vi "plotFrd.vi"(8 "error in (no error)":errorcluster, 9 "FRD-array":T1[](array[typedef]), 10 "Phase Graph Reference in":refnum<vi>, 11 "Magnitude Graph Reference in":refnum<vi>) -> (0 "error out":errorcluster, 2 "Phase Graph Reference out":refnum<vi>, 3 "Magnitude Graph Reference out":refnum<vi>)   [LabVIEW 2017]
uses:
  auto-sys-id/controls/FrdData.ctl
  <vilib>/Analysis/NI_AALPro.lvlib
panel:
  in  "Frequency Unit":enum16{"Hz", "rad/s"}(ring)
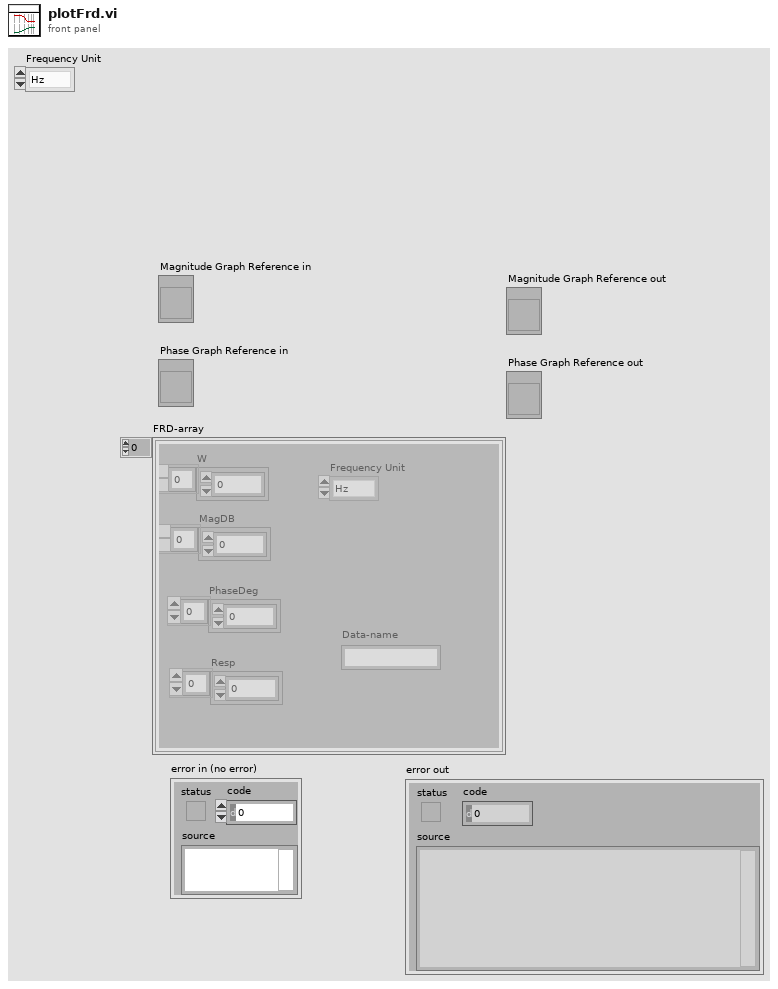
[diagram p1: front panel]
types:
  T1 = typedef "FrdData.ctl" = cluster{"Frequency Unit":enum16{"Hz", "rad/s"}, "W":dbl[], "MagDB":dbl[], "PhaseDeg":dbl[], "Resp":cdb[], "Data-name":string}
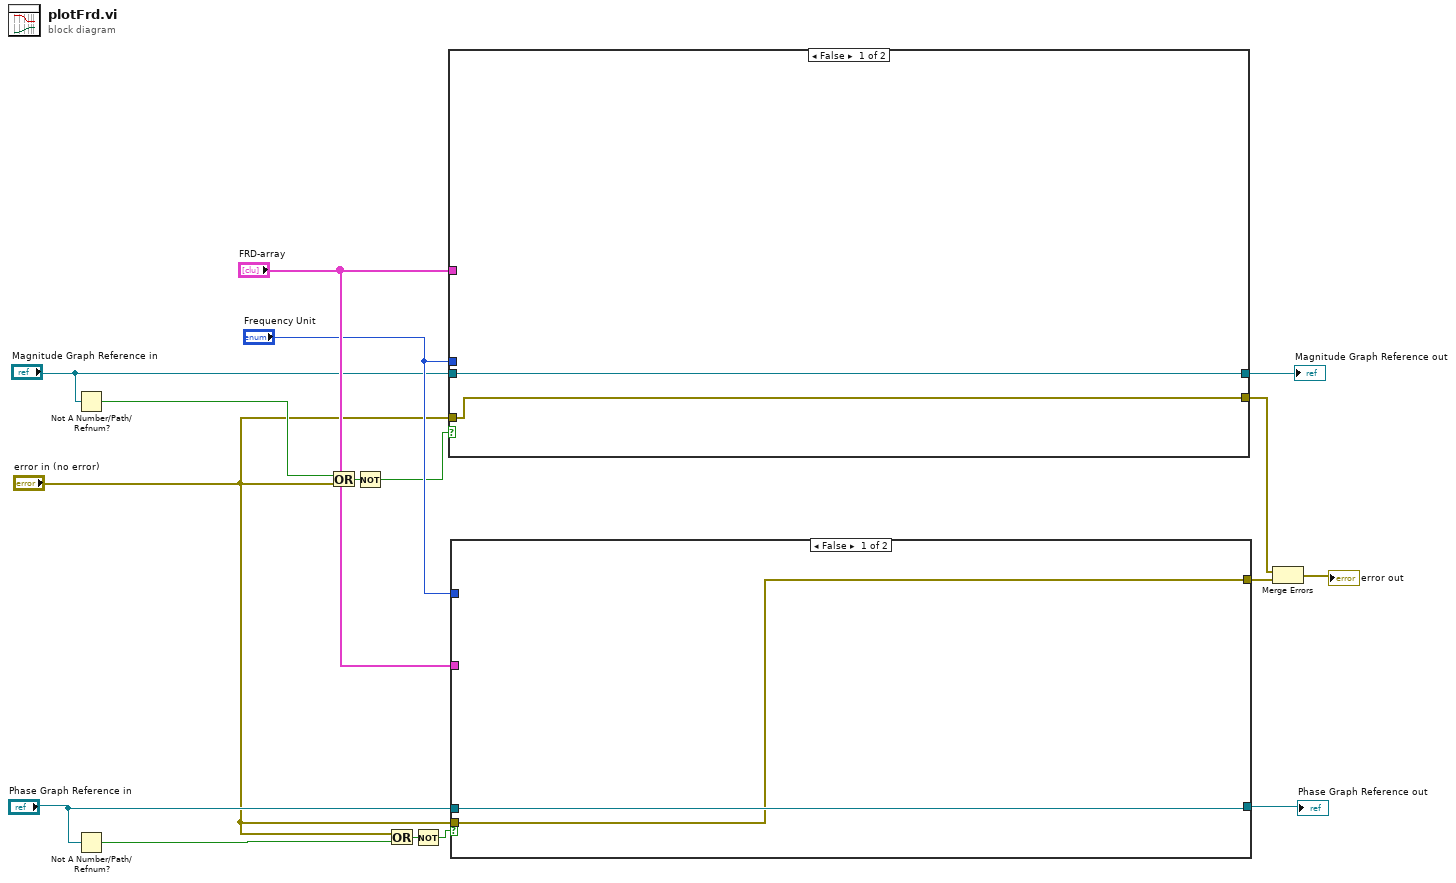
[diagram p0: block diagram]
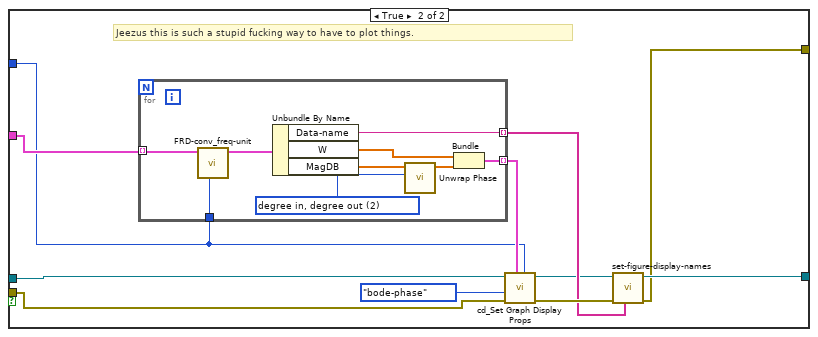
[diagram p2: hidden frame]
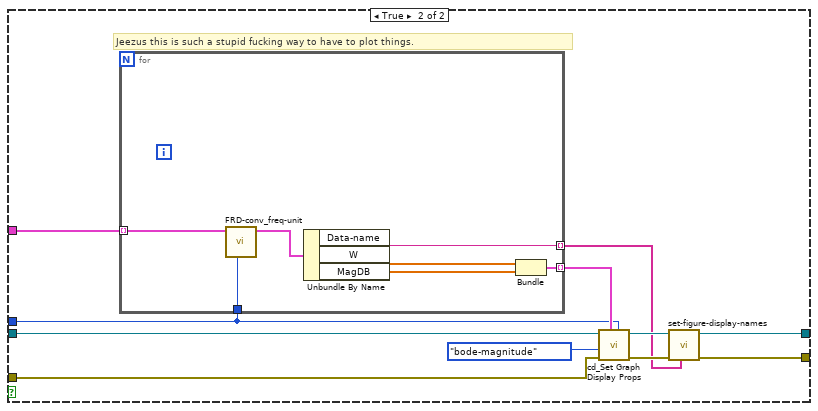
[diagram p3: hidden frame]
diagram:
  n1 = Not A Number/Path/Refnum?(number/path/refnum="Magnitude Graph Reference in") -> (NaN/Path/Refnum?=w2:bool)
  n2 = Not A Number/Path/Refnum?(number/path/refnum="Phase Graph Reference in") -> (NaN/Path/Refnum?=w7:bool)
  n3 = Or(x=w2, y="error in (no error)") -> (x .or. y?=w4:bool)
  n4 = Not(x=w4) -> (.not. x?=w3:bool)
  n5 = Or(x="error in (no error)", y=w7) -> (x .or. y?=w5:bool)
  n6 = Not(x=w5) -> (.not. x?=w6:bool)
  n7 = case shown="False" w3 {
    tunnel: "Magnitude Graph Reference in" -> [w18 w29]
    tunnel: [w18 w22] -> w16
    tunnel: [w17 w24] -> w13
    tunnel: "FRD-array" -> [_ w26]
    tunnel: "Frequency Unit" -> [_ w20]
    tunnel: "error in (no error)" -> [w17 w19]
    frame False {
    }
    frame True {
      # "Jeezus this is such a stupid fucking way to have to plot things."
      n8 = for {
        tunnel: [w35] -> w27 mode=indexing
        tunnel: w26 -> [w34] mode=indexing
        tunnel: [w30] -> w21 mode=indexing
        tunnel: w20 -> [w33]
        n9 = call "FRD-conv_freq-unit.vi"("Frequency Unit"=w33, "FRD-model"=w34) -> ("FRD-out"=w32:T1)  [unwired: 9 in]
        n10 = Unbundle By Name(w32) -> ("Data-name"=w30:string, "W"=w31:dbl[], "MagDB"=w36:dbl[])
        n11 = Bundle("W"=w31, "MagDB"=w36) -> (w35:cluster{"W":dbl[], "MagDB":dbl[]})  [unwired: 1 in]
      }
      n12 = call <vilib>:"cd_Set Graph Display Props.vi"("Frequency Unit"=w20, "Plots"=w27, "error in (no error)"=w19, "plot type"=enum16{"bode-magnitude", "bode-phase"}."bode-magnitude", "Graph Ref In"=w29) -> ("error out"=w25:errorcluster, "Graph Ref out"=w23:refnum<vi>)  [unwired: 3 in, 2 out]
      n13 = call "set-figure-display-names.vi"("DisplayNames"=w21, "error in"=w25, "figure (in)"=w23) -> ("error out"=w24:errorcluster, "figure (out)"=w22:refnum<vi>)  [unwired: 7 in]
    }
  }
  "Magnitude Graph Reference out" <- w16
  n14 = case shown="False" w6 {
    tunnel: "Phase Graph Reference in" -> [w38 w49]
    tunnel: [w38 w45] -> w15
    tunnel: "FRD-array" -> [_ w46]
    tunnel: [w37 w39] -> w14
    tunnel: "Frequency Unit" -> [_ w41]
    tunnel: "error in (no error)" -> [w37 w40]
    frame False {
    }
    frame True {
      # "Jeezus this is such a stupid fucking way to have to plot things."
      n15 = for {
        tunnel: [w58] -> w47 mode=indexing
        tunnel: w46 -> [w51] mode=indexing
        tunnel: [w53] -> w43 mode=indexing
        tunnel: w41 -> [w50]
        w56 = 2 items=["radian in, radian out", "radian in, degree out", "degree in, degree out", "degree in, radian out"] ("phase unit")
        n16 = call "FRD-conv_freq-unit.vi"("Frequency Unit"=w50, "FRD-model"=w51) -> ("FRD-out"=w52:T1)  [unwired: 9 in]
        n17 = Unbundle By Name(w52) -> ("Data-name"=w53:string, "W"=w55:dbl[], "MagDB"=w54:dbl[])
        n18 = call <vilib>:"Unwrap Phase.vi"("phase unit"=w56, "Phase"=w54) -> ("Unwrapped Phase"=w57:dbl[])  [unwired: 8 in, 1 out]
        n19 = Bundle("W"=w55, "Unwrapped Phase"=w57) -> (w58:cluster{"W":dbl[], "Unwrapped Phase":dbl[]})  [unwired: 1 in]
      }
      n20 = call <vilib>:"cd_Set Graph Display Props.vi"("Frequency Unit"=w41, "Plots"=w47, "error in (no error)"=w40, "plot type"=enum16{"bode-magnitude", "bode-phase"}."bode-phase", "Graph Ref In"=w49) -> ("error out"=w44:errorcluster, "Graph Ref out"=w42:refnum<vi>)  [unwired: 3 in, 2 out]
      n21 = call "set-figure-display-names.vi"("DisplayNames"=w43, "error in"=w44, "figure (in)"=w42) -> ("error out"=w39:errorcluster, "figure (out)"=w45:refnum<vi>)  [unwired: 7 in]
    }
  }
  "Phase Graph Reference out" <- w15
  n22 = Merge Errors(w13, w14) -> (→"error out":errorcluster)
